vi "Main.vi"() -> ()   [LabVIEW 2024, in "UI.lvlib"]
uses:
  UI.lvlib
  UI_Model/state_app.ctl
panel:
  in  "stop":bool
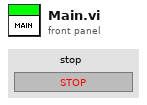
[diagram p1: front panel]
types:
  T1 = typedef "UI.lvlib/state_app.ctl" = enum16{"Init", "Stop"}
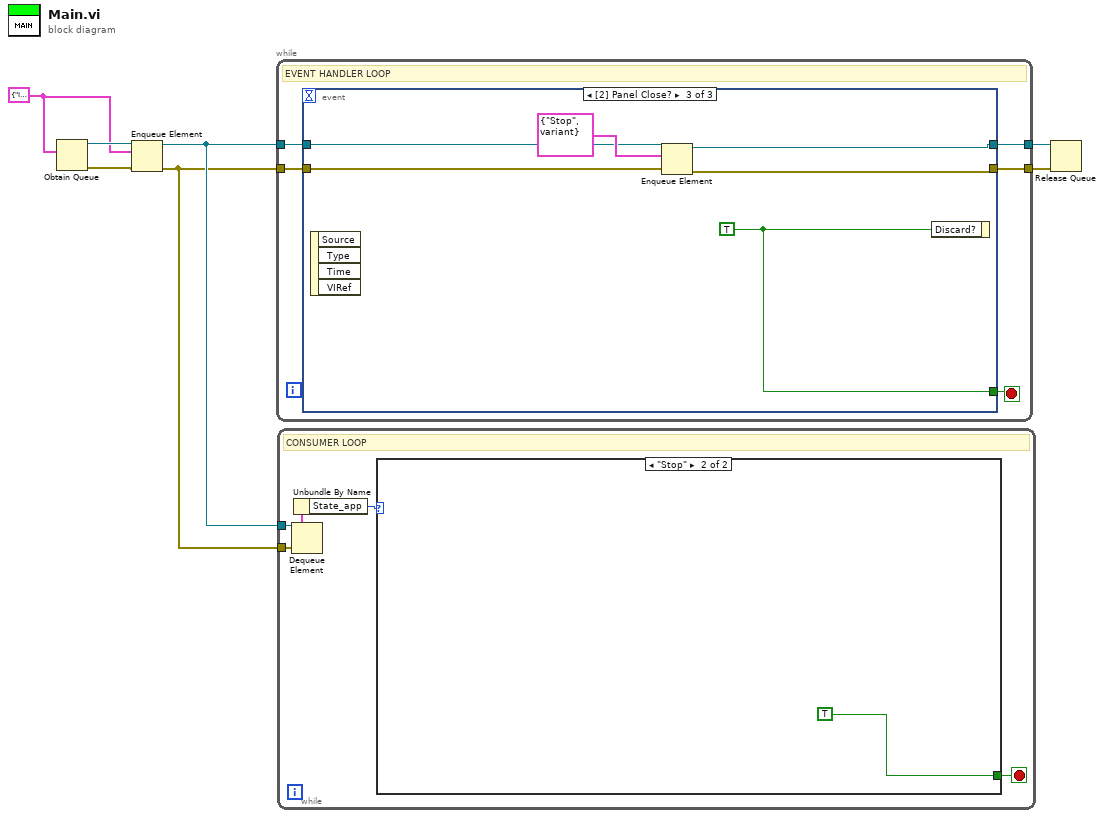
[diagram p0: block diagram]
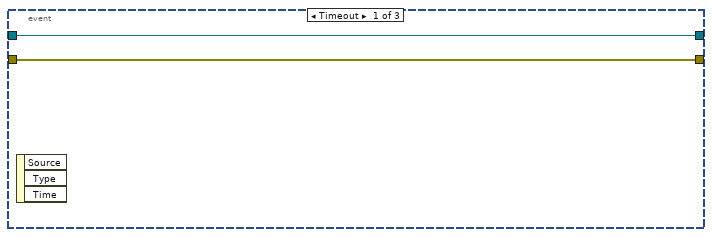
[diagram p3: hidden frame]
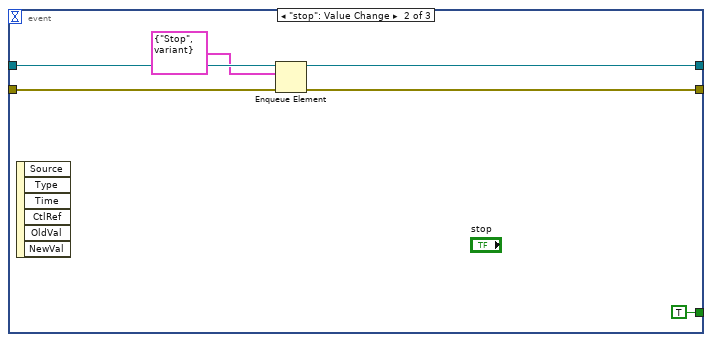
[diagram p4: hidden frame]
diagram:
  w1 = cluster{"State_app":T1, "Data":variant} {"State_app"=enum."Init", "Data"=variant}
  n1 = Obtain Queue(element data type=w1) -> (queue out=w7:refnum<queue>, error out=w6:errorcluster)  [unwired: 4 in, 1 out]
  n2 = Enqueue Element(queue=w7, element=w1, error in (no error)=w6) -> (queue out=w3:refnum<queue>, error out=w2:errorcluster)  [unwired: 1 in, 1 out]
  n3 = while {
    tunnel: w3 -> [w11]
    tunnel: w2 -> [w10]
    tunnel: [w9] -> w4
    tunnel: [w8] -> w5
    stop <- w12 stop-if-true
    # "EVENT HANDLER LOOP"
    n4 = event shown="[2] Panel Close?" {
      selector: _ -> [_ _ _]
      dyn-events: _ -> [_ _ _]
      timeout: _ -> [_ _ _]
      tunnel: [_ TRUE ("Discard?") w26] -> w12
      tunnel: w11 -> [w14 w19 w23]
      tunnel: w10 -> [w13 w20 w24]
      tunnel: [w14 w17 w21] -> w8
      tunnel: [w13 w16 w22] -> w9
      event Timeout {
        n5 = event-data() -> ()  [unwired: 1 in, 3 out]
      }
      event "stop": Value Change {
        n6 = event-data() -> ()  [unwired: 1 in, 6 out]
        n7 = Enqueue Element(queue=w19, element=cluster{"State_app":T1, "Data":variant} {"State_app"=enum."Stop", "Data"=variant}, error in (no error)=w20) -> (queue out=w17:refnum<queue>, error out=w16:errorcluster)  [unwired: 1 in, 1 out]
      }
      event Panel Close? {
        w26 = TRUE ("Discard?")
        n8 = event-data() -> ()  [unwired: 1 in, 4 out]
        n9 = Enqueue Element(queue=w23, element=cluster{"State_app":T1, "Data":variant} {"State_app"=enum."Stop", "Data"=variant}, error in (no error)=w24) -> (queue out=w21:refnum<queue>, error out=w22:errorcluster)  [unwired: 1 in, 1 out]
        n10 = event-data("Discard?"=w26) -> ()  [unwired: 1 in, 1 out]
      }
    }
  }
  n11 = while {
    tunnel: w3 -> [w30]
    tunnel: w2 -> [w31]
    stop <- w27 stop-if-true
    # "CONSUMER LOOP"
    n12 = Dequeue Element(queue=w30, error in (no error)=w31) -> (element=w29:cluster{"State_app":T1, "Data":variant})  [unwired: 1 in, 3 out]
    n13 = Unbundle By Name(w29) -> ("State_app"=w28:T1)
    n14 = case shown="\"Stop\"" w28 {
      tunnel: [_ TRUE] -> w27
      frame "Init", Default {
      }
      frame "Stop" {
      }
    }
  }
  n15 = Release Queue(queue=w5, error in (no error)=w4) -> ()  [unwired: 1 in, 3 out]
